vi "goback.vi"(2 "NXT/EV3":T1) -> (0 "NXT/EV3 2":T1)   [LabVIEW 2016]
uses:
  <vilib>/NXT/Subs/LVHSConnector.ctl
  <vilib>/NXT/LegoClasses/BrickReference/BrickReference.lvclass
  <vilib>/NXT/Block Support/NXT_InputPort.ctl
  <vilib>/NXT/Block Support/NXT_OutputPort.ctl
  <vilib>/NXT/NXTIO Xnodes/NXTIONodeSubVIs/NXTMoveMotors.vi
  <vilib>/NXT/Dual Mode Library/Waits/Wait_Touch.vi
  <vilib>/NXT/NXTIO Xnodes/NXTIONodeSubVIs/NXTStopMotors.vi
  <vilib>/NXT/NXTIO Xnodes/AddressXNode/NXTIOAddress.xnode
  <vilib>/NXT/NXTIO Xnodes/NXTIOXNode/NXTIO.xnode
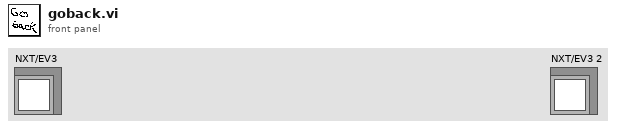
[diagram p1: front panel]
types:
  T1 = typedef "LVHSConnector.ctl" = refnum<class "BrickReference.lvclass">
  T2 = typedef "NXT_InputPort.ctl" = u32
  T3 = typedef "NXT_OutputPort.ctl" = u8
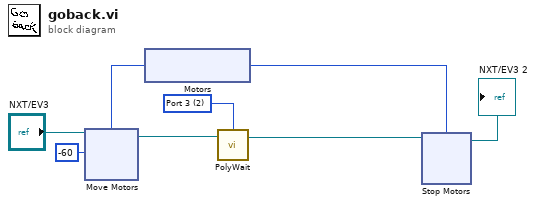
[diagram p0: block diagram]
diagram:
  w3 = T2 2 items=["Port 1", "Port 2", "Port 3", "Port 4"] ("Port (Port 1)")
  n1 = xnode "Motors"() -> ("Motor"=w2:T3)
  n2 = xnode "Move Motors"("Power/Speed 1"=i8 -60, "Motors"=w2, "NXT/EV3"="NXT/EV3") -> ("NXT/EV3"=w5:T1)
  n3 = call-poly <vilib>:"PolyWait.vi"("NXT/EV3"=w5, "Port (Port 1)"=w3) -> ("NXT/EV3"=w4:T1)  [unwired: 2 in]
  n4 = xnode "Stop Motors"("Motors"=w2, "NXT/EV3"=w4) -> ("NXT/EV3"=→"NXT/EV3 2":T1)
